vi "SVFA Power in Band (1 Ch).vi"(0 "spectrum":cluster{"x0":dbl, "dx":dbl, "magnitude":dbl[]} {"magnitude" format="%.2f"; "dx" format="%.2f"; "x0" format="%.2f"}, 1 "range":cluster{"start":dbl, "stop":dbl}={"start"=-1.0, "stop"=-1.0} {"stop" format="%.2f"; "start" format="%.2f"}, 4 "spectrum info":T1={"channel name"="", "description"="", "x-axis units"=0, "spectral info"={"spectrum type"=enum."Power [Magnitude^2]", "linear/dB"=enum."linear", "window"=0, "window size"=0, "FFT size"=0}, "engineering units"=0, "custom label"="", "dB reference [EU]"=0.0, "peak units"=enum."rms", "weighting filter"=0, "spectral density?"=FALSE, "unit label"="", "spectrum skewed?"=FALSE, "complimentary spectrum units"=enum."none"} {"x-axis units" items=["Time (s)"=0, "Frequency-CB (Hz)"=1, "Frequency-CPB (Hz)"=1248, "Frequency-Arbitrary (Hz)"=2357, "Quefrency (s)"=2, "Revolutions (rev)"=3, "Order"=4, "Speed (RPM)"=11, "Speed (rad/s)"=21, "Index"=65535]; "weighting filter" items=["Linear", "A-weighting", "B-weighting", "C-weighting", "ITU-R 468-4", "Dolby", "CCITT", "C-message", "Wb", "Wc", "Wd", "We", "Wf", "Wh", "Wj", "Wk", "Wm", "AES17 20 kHz lowpass", "AES17 40 kHz lowpass", "AES17 20 kHz highpass", "AES17 40 kHz highpass"]; "dB reference [EU]" format="%.2f"; "engineering units" items=["custom..."=0, "V"=1, "A"=21, "C"=30, "pC"=31, "s"=32, "-"=29, "Pa"=2, "N"=20, "g"=3, "m/s^2"=4, "m/s"=5, "m"=6, "mm/s"=12, "mm"=13, "micron/s"=14, "micron"=15, "in/s^2"=7, "in/s"=8, "in"=9, "mil/s"=10, "mil"=11, "rad/s^2"=16, "rad/s"=17, "rad"=18, "deg/s^2"=26, "deg/s"=27, "deg"=28, "RPM"=22, "cycle/s^2"=23, "Hz"=24, "cycle"=25, "strain"=19]; "spectral info"."window" items=["None "=0, "Hanning"=1, "Hamming"=2, "Blackman-Harris"=3, "Exact Blackman"=4, "Blackman"=5, "Flat Top"=6, "4 Term B-Harris "=7, "7 Term B-Harris"=8, "Low Sidelobe"=9, "Force - Exponential"=10, "Gaussian"=62]}, 5 "error in (no error)":errorcluster) -> (14 "power in band":dbl=nan format="%.2f", 15 "unit label":string, 19 "error out":errorcluster)   [LabVIEW 2017]
doc: "Computes the aggregate power in the <B>range</B>. The SVFA Power in Band VI operates on Power, PSD, COP, and FFT [Mag] spectra. Wire data to the <B>spectrum</B> input to determine the polymorphic instance to use or manually select the instance."
uses:
  <vilib>/addons/_NISVFA/_Shared subVIs/Controls/svc_Spectrum Info.ctl
  <vilib>/addons/_NISVFA/_Shared subVIs/Controls/svc_X-Axis Units.ctl
  <vilib>/addons/_NISVFA/_Shared subVIs/Controls/svc_Spectrum Type.ctl
  <vilib>/addons/_NISVFA/_Shared subVIs/Controls/svc_Engineering Units Text Ring.ctl
  <vilib>/addons/_NISVFA/_Shared subVIs/Controls/svc_Weighting Filter Text Ring.ctl
  <vilib>/addons/_NISVFA/_Shared subVIs/Controls/svc_Complimentary Spectrum Units.ctl
  <vilib>/addons/_NISVFA/_Spectrum Processing/SVFA Get Spectrum Subset (1 Ch).vi
  <vilib>/addons/_NISVFA/_Spectrum Processing/SVFA Unit Conversion (1 Ch).vi
  <vilib>/addons/_NISVFA/_Spectrum Processing/subVIs/svfa_Conversion Utility (spectrum info).vi
  <vilib>/addons/_NISVFA/_Spectrum Processing/subVIs/svfa_Peak to RMS to Peak2Peak.vi
  <vilib>/addons/_NISVFA/_Spectrum Processing/subVIs/svfa_Mag to Mag2.vi
  <vilib>/addons/_NISVFA/_Spectrum Processing/subVIs/svfa_Linear to dB.vi
  <vilib>/addons/_NISVFA/_Spectrum Processing/subVIs/svfa_dBrefA to dBrefB.vi
  <vilib>/addons/_NISVFA/_Spectrum Processing/subVIs/svfa_Spectrum to Spectral Density.vi
  <vilib>/addons/_NISVFA/_Shared subVIs/Common/svc_Get Weighting Enum and Labels.vi
  <vilib>/addons/_NISVFA/_Shared subVIs/Common/svc_Unit Label Lexical Class.vi
  <vilib>/addons/_NISVFA/_Shared subVIs/Common/svc_Engineering Units to Unit Label.vi
  <vilib>/addons/_NISVFA/_Shared subVIs/Common/svc_Format Value (DBL).vi
  <vilib>/addons/_NISVFA/_Shared subVIs/Common/svc_Build Unit Label for Frequency Range.vi
  <vilib>/addons/_NISVFA/_Shared subVIs/Common/svc_Convert Frequency to Frequency String.vi
  <vilib>/addons/_NISVFA/_Shared subVIs/Common/svc_Check Frequency Range in Spectrum.vi
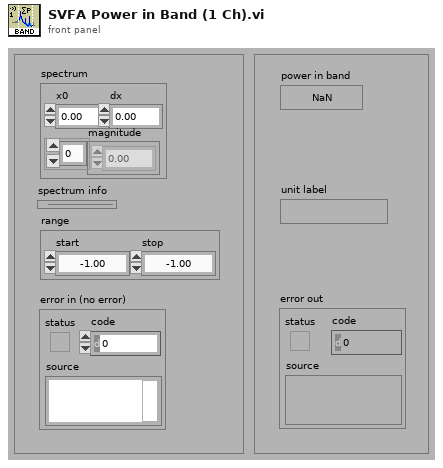
[diagram p1: front panel]
types:
  T1 = typedef "svc_Spectrum Info.ctl" = cluster{"channel name":string, "description":string, "x-axis units":T2, "spectral info":cluster{"spectrum type":T3, "linear/dB":enum16{"linear", "dB"}, "window":u16, "window size":i32, "FFT size":i32}, "engineering units":T4, "custom label":string, "dB reference [EU]":dbl, "peak units":enum16{"rms", "peak", "peak-peak"}, "weighting filter":T5, "spectral density?":bool, "unit label":string, "spectrum skewed?":bool, "complimentary spectrum units":T6}
  T2 = typedef "svc_X-Axis Units.ctl" = u16
  T3 = typedef "svc_Spectrum Type.ctl" = enum16{"FFT Spectrum [complex]", "Amplitude [Magnitude]", "Power [Magnitude^2]", "Cross Spectrum [complex]", "Frequency Response [Complex]"}
  T4 = typedef "svc_Engineering Units Text Ring.ctl" = u16
  T5 = typedef "svc_Weighting Filter Text Ring.ctl" = u16
  T6 = typedef "svc_Complimentary Spectrum Units.ctl" = enum16{"none", "radians", "degrees", "cycles", "imaginary"}
  T7 = enum16{"no change", "spectrum", "spectral density"}
  T8 = cluster{"linear/dB":enum16{"no change", "linear", "dB"}, "dB reference (0: no change)":dbl, "power/magnitude":enum16{"no change", "power", "magnitude"}, "view":enum16{"no change", "rms", "peak", "peak-peak"}}
  T9 = typedef "NI_AALPro.lvlib/windowTd.ctl" = u32
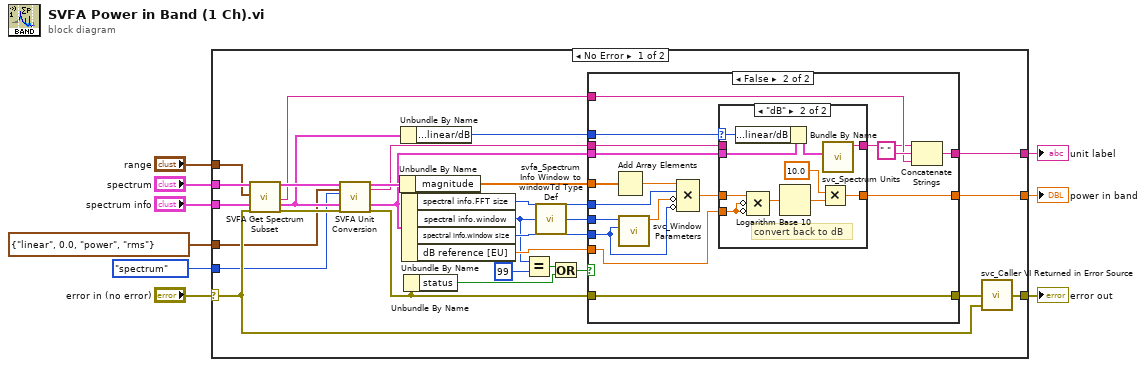
[diagram p0: block diagram]
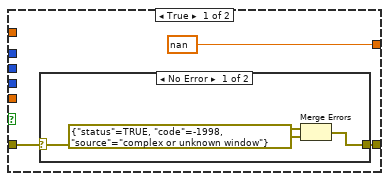
[diagram p2: hidden frame]
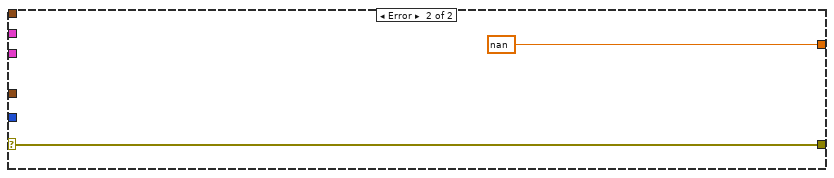
[diagram p5: hidden frame]
diagram:
  n1 = case shown="No Error" "error in (no error)" {
    selector: "error in (no error)" -> [w36 w76]
    tunnel: "spectrum" -> [w35 _]
    tunnel: [w34 nan ("power in band")] -> w8
    tunnel: [w38 w76] -> w7
    tunnel: "range" -> [w33 _]
    tunnel: "spectrum info" -> [w37 _]
    tunnel: [w21 _] -> w4
    tunnel: T8 {"linear/dB"=enum."linear", "dB reference (0: no change)"=0.0, "power/magnitude"=enum."power", "view"=enum."rms"} ("desired scaling") -> [w12 _]
    tunnel: T7."spectrum" ("spectral density desired") -> [w11 _]
    frame No Error {
      n2 = call-poly <vilib>:"SVFA Get Spectrum Subset.vi"("spectrum"=w35, "range"=w33, "spectrum info"=w37, "error in (no error)"=w36) -> ("spectrum subset"=w31:cluster{"x0":dbl, "dx":dbl, "magnitude":dbl[]}, "range label"=w22:string, "dup spectrum info"=w14:T1, "error out"=w29:errorcluster)  [unwired: 10 in, 2 out]
      n3 = call-poly <vilib>:"SVFA Unit Conversion.vi"("spectrum"=w31, "desired scaling"=w12, "spectral density desired"=w11, "spectrum info in"=w14, "error in (no error)"=w29) -> ("converted spectrum"=w30:cluster{"x0":dbl, "dx":dbl, "magnitude":dbl[]}, "unit label"=w13:string, "spectrum info out"=w23:T1, "error out"=w17:errorcluster)  [unwired: 11 in]
      n4 = Unbundle By Name(w30) -> ("magnitude"=w32:dbl[])
      n5 = Unbundle By Name(w14) -> ("spectral info.linear/dB"=w25:enum16{"linear", "dB"})
      n6 = Unbundle By Name(w23) -> ("spectral info.FFT size"=w27:i32, "spectral info.window"=w19:u16, "spectral info.window size"=w28:i32, "dB reference [EU]"=w26:dbl)
      n7 = Unbundle By Name(w17) -> ("status"=w16:bool)
      n8 = Equal?(x=w19, y=u16 99) -> (x = y?=w20:bool)
      n9 = call <vilib>:"svfa_Spectrum Info Window to windowTd Type Def.vi"("window"=w19) -> ("window"=w10:T9)  [unwired: 4 in]
      n10 = Or(x=w20, y=w16) -> (x .or. y?=w15:bool)
      n11 = case shown="False" w15 {
        tunnel: [nan w62] -> w34
        tunnel: w32 -> [_ w61]
        tunnel: w17 -> [w39 w47]
        tunnel: [w41 w47] -> w24
        tunnel: w28 -> [_ w60]
        tunnel: w27 -> [_ w59]
        tunnel: w26 -> [_ w55]
        tunnel: w25 -> [_ w54]
        tunnel: [_ w50] -> w21
        tunnel: w23 -> [_ w53]
        tunnel: w22 -> [_ w51]
        tunnel: w10 -> [_ w49]
        tunnel: w13 -> [_ w46]
        frame True {
          n12 = case shown="No Error" w39 {
            selector: w39 -> [w42 w45]
            tunnel: [w43 w45] -> w41
            frame No Error {
              n13 = Merge Errors(w42, errorcluster {"status"=TRUE, "code"=-1998, "source"="complex or unknown window"} ("error out")) -> (w43:errorcluster)
            }
            frame Error {
            }
          }
        }
        frame False {
          n14 = Add Array Elements(numeric array=w61) -> (sum=w57:dbl)
          n15 = call <vilib>:"svc_Window Parameters.vi"("window size"=w60, "window"=w49) -> ("ENBW"=w56:dbl)  [unwired: 6 in, 3 out]
          n16 = Compound Arithmetic op=MULTIPLY(w57, w59, invert w56, invert w60) -> (w58:dbl)
          n17 = case shown="\"dB\"" w54 {
            selector: w54 -> [_ w68]
            tunnel: [w64 w74] -> w62
            tunnel: w58 -> [w64 w70]
            tunnel: w55 -> [_ w71]
            tunnel: w53 -> [_ w67]
            tunnel: [w63 w65] -> w48
            tunnel: w46 -> [w63 _]
            frame "linear", Default {
            }
            frame "dB" {
              # "convert back to dB"
              n18 = Bundle By Name(cluster=w67, "spectral info.linear/dB"=w68) -> (w66:T1)
              n19 = Compound Arithmetic op=MULTIPLY(w70, invert w71, invert w71) -> (w69:dbl)
              n20 = Logarithm Base 10(1:w69) -> (0:w73:dbl)
              n21 = Multiply(x=10.0 ("Numeric"), y=w73) -> (x*y=w74:dbl)
              n22 = call <vilib>:"svc_Spectrum Units.vi"("spectrum info in"=w66) -> ("unit label"=w65:string)  [unwired: 3 in, 3 out]
            }
          }
          n23 = Concatenate Strings(w48, " " ("string"), w51) -> (w50:string)
        }
      }
      n24 = call <vilib>:"svc_Caller VI Returned in Error Source.vi"("warning input to caller"=w36, "error in (no error)"=w24) -> ("error out"=w38:errorcluster)  [unwired: 3 in]
    }
    frame Error {
    }
  }
  "error out" <- w7
  "power in band" <- w8
  "unit label" <- w4
